vi "sexto.vi"() -> ()   [LabVIEW 2012]
panel:
  in  "Numeric":dbl
  in  "stop":bool
  out "Resultado":dbl
  in  "Dato 2":dbl
  in  "Dato1":dbl
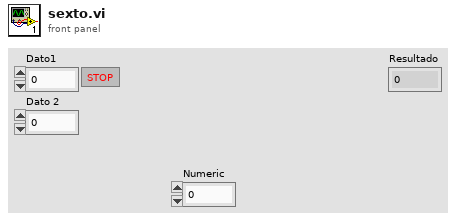
[diagram p1: front panel]
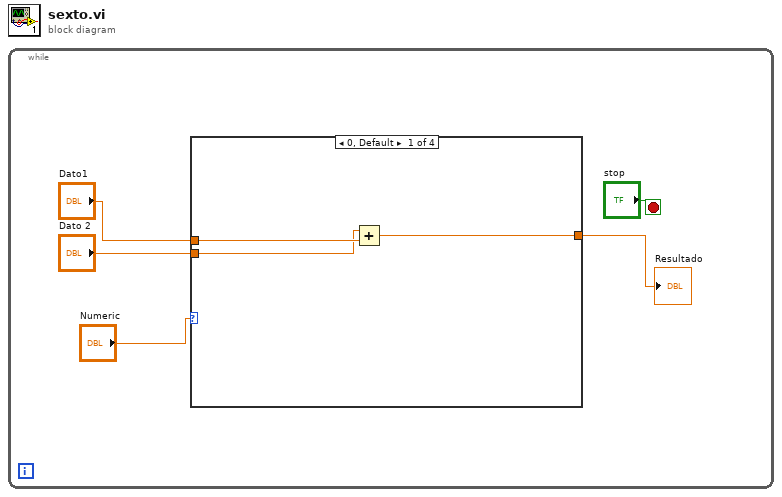
[diagram p0: block diagram]
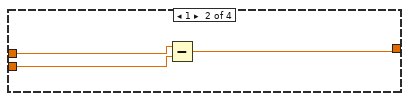
[diagram p2: hidden frame]
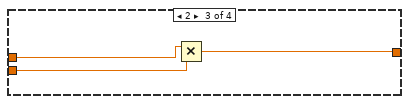
[diagram p3: hidden frame]
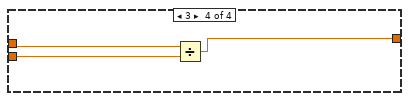
[diagram p4: hidden frame]
diagram:
  n1 = while {
    stop <- "stop" stop-if-true
    n2 = case shown="0, Default" "Numeric" {
      tunnel: "Dato1" -> [w8 w11 w14 w17]
      tunnel: "Dato 2" -> [w7 w10 w13 w16]
      tunnel: [w6 w9 w12 w15] -> w3
      frame 0, Default {
        n3 = Add(x=w7, y=w8) -> (x+y=w6:dbl)
      }
      frame 1 {
        n4 = Subtract(x=w11, y=w10) -> (x-y=w9:dbl)
      }
      frame 2 {
        n5 = Multiply(x=w14, y=w13) -> (x*y=w12:dbl)
      }
      frame 3 {
        n6 = Divide(x=w17, y=w16) -> (x/y=w15:dbl)
      }
    }
    "Resultado" <- w3
  }
